vi "_REF_.vi"(0 "System no.":i32=1 min=1 max=4 step=1, 2 "Axes to query":string[](array[string]), 3 "All axes?":bool, 4 "Axis identifier?":bool=TRUE, 5 "error in":errorcluster) -> (14 "Axis with reference?":bool[](array[boolean]), 19 "error out":errorcluster)   [LabVIEW 2012]
doc: "Indicates whether queried axes have a reference switch or not.\n\nValid for C-702, C-843, C-843.PM, C-844, C-848, C-865, C-866, C-880, C-880K005, Mercury\n\nC-702: If All axes = TRUE, then Axis identifier can be FALSE\nC-843: If All axes = TRUE, then Axis identifier must be TRUE\nC-843.PM: If All axes = TRUE, then Axis identifier must be TRUE\nC-844: If All axes = TRUE, then Axis identifier must be TRUE\nC-848: If All axes = TRUE, then Axis identifier can be FALSE\nC-865: If All axes = TRUE, then Axis identifier must be TRUE\nC-866: If All axes = TRUE, then Axis identifier must be TRUE\nC-880: If All axes = TRUE, then Axis identifier can be FALSE\nC-880K005: VI only supported when called through PI_Multix.vi\nMercury: If All axes = TRUE, then Axis identifier can be FALSE"
panel:
  # "Indicates whether queried axes have a reference switch or not."
  # "If all axes: use"
  # "Query"
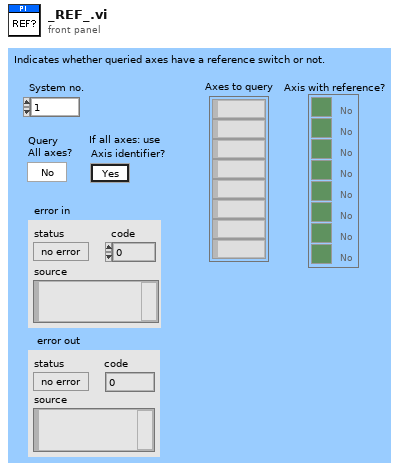
[diagram p1: front panel]
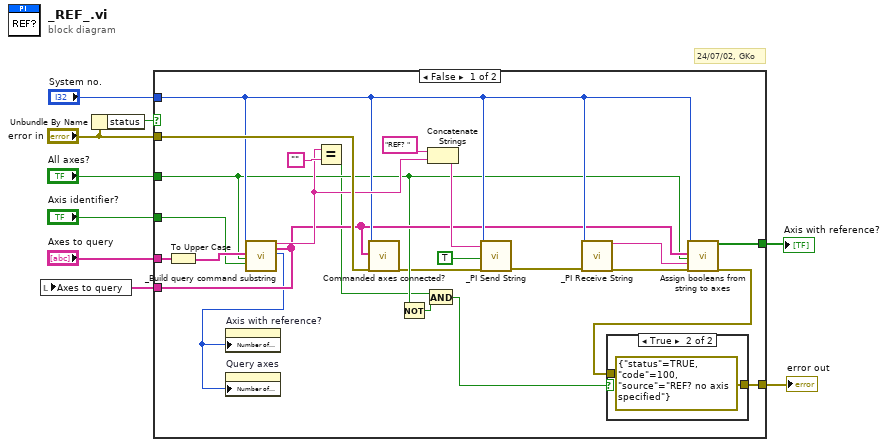
[diagram p0: block diagram]
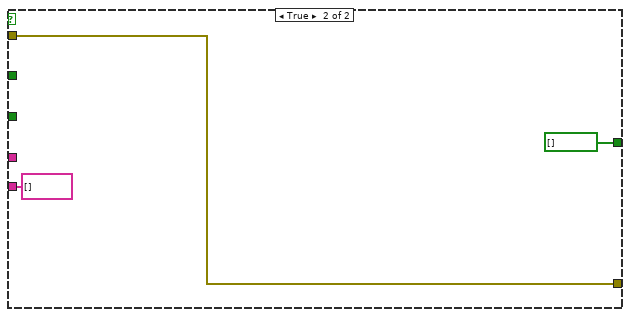
[diagram p3: hidden frame]
diagram:
  # "24/07/02, GKo"
  n1 = Unbundle By Name("error in") -> ("status"=w2:bool)
  n2 = case shown="False" w2 {
    tunnel: [w28 bool[] [] ("Booleans")] -> w9
    tunnel: "error in" -> [w27 w37]
    tunnel: "Axes to query" -> [w26 _]
    tunnel: [w23 w37] -> w7
    tunnel: "Axis identifier?" -> [w21 _]
    tunnel: "System no." -> [w19 _]
    tunnel: [w18 string[] [] ("Axes to query out")] -> w4
    tunnel: "All axes?" -> [w17 _]
    frame False {
      n3 = To Upper Case(1:w26) -> (0:w22:string[])
      n4 = call "_Build query command substring.vi"("System no."=w19, "Axes to query in"=w22, "Query\nAll axes?"=w17, "For all axes: use\nAxis identifier?"=w21) -> ("Command substring"=w20:string, "Axes to query out"=w18:string[], "Number of rows"=w12:u32)  [unwired: 13 in]
      n5 = property on="Axis with reference?" class="Arr (strict)"("Number of Rows"=w12) -> ()  [unwired: 2 in, 2 out]
      n6 = property on="Query axes" class="Arr (strict)"("Number of Rows"=w12) -> ()  [unwired: 2 in, 2 out]
      n7 = Equal?(x=w20, y="" ("x")) -> (x = y?=w14:bool)
      n8 = call "Commanded axes connected?.vi"("System no."=w19, "Commanded axes"=w18, "error in"=w27) -> ("error out"=w11:errorcluster)  [unwired: 15 in, 1 out]
      n9 = Not(x=w17) -> (.not. x?=w13:bool)
      n10 = And(x=w14, y=w13) -> (x .and. y?=w24:bool)
      n11 = Concatenate Strings("REF? ", w20) -> (w29:string)
      n12 = call "_PI Send String.vi"("System no."=w19, "String to send"=w29, "Attach termination char.?"=TRUE ("Attach Linefeed?"), "error in"=w11) -> ("error out"=w32:errorcluster)  [unwired: 15 in]
      n13 = call "_PI Receive String.vi"("System no."=w19, "error in"=w32) -> ("String read"=w16:string, "error out"=w10:errorcluster)  [unwired: 15 in, 1 out]
      n14 = call "Assign booleans from string to axes.vi"("System no."=w19, "Queried axes"=w18, "All axes queried?"=w17, "Input String"=w16, "error in"=w10) -> ("Booleans"=w28:bool[], "error out"=w15:errorcluster)  [unwired: 13 in]
      n15 = case shown="True" w24 {
        tunnel: [w33 errorcluster {"status"=TRUE, "code"=100, "source"="REF? no axis specified"} ("error out")] -> w23
        tunnel: w15 -> [w33 _]
        frame False {
        }
        frame True {
        }
      }
    }
    frame True {
    }
  }
  "error out" <- w7
  "Axis with reference?" <- w9
  n16 = local write "Axes to query"(w4) -> ()
